vi "WzNetRem_Example_General.vi"() -> ()   [LabVIEW 2012]
uses:
  Wizzler_NetworkRemoteToolkit.lvlib
panel:
  out "Signal Goodness":cluster{"Value":dbl, "Warning":string} {"Value" scale=0.9..2.0}
  out "Signal Level":cluster{"Value":dbl, "Warning":string} {"Value" scale=0.0..65535.0}
  out "Time profile":cluster{"Time":dbl[], "Intensity":dbl[]}[](graph)
  out "Numerics":T1={"Autoco duration FWHM"=0.0, "FTL time width FWHM"=nan, "TBP FWHM"=nan, "Spectral width FWHM"=nan, "Time width FWHM"=nan, "Mean wavelength"=nan, "Time stand. dev."=nan, "FTL time stand. dev."=nan, "Mean freq"=nan, "Spectral stand. dev."=nan, "TBP stand. dev."=nan, "Spectral width FWHM - nu"=nan, "Spectral stand. dev. - nu"=nan} {"Spectral stand. dev. - nu" format="%#.1f"; "Spectral width FWHM - nu" format="%#.1f"; "TBP stand. dev." format="%#.3f"; "Spectral stand. dev." format="%#.1f"; "Mean freq" format="%#.1f"; "FTL time stand. dev." format="%#.1f"; "Time stand. dev." format="%#.1f"; "Mean wavelength" format="%#.1f"; "Time width FWHM" format="%#.1f"; "Spectral width FWHM" format="%#.1f"; "TBP FWHM" format="%#.3f"; "FTL time width FWHM" format="%#.1f"}
  in  "stop":bool
  in  "New Status":T2={"New Algorithm"=1, "Integration Time"=0.002, "LambdaMin"=7e-07, "LambdaMax"=9e-07} {"New Algorithm" items=["Spectrum", "SRSI"]}
  out "Previous Status":T3
  out "error out":errorcluster
  out "Time Stamp":string
  out "Spectral Data":cluster{"Frequencies":ext[], "Phase":dbl[]}[](graph)
  in  "machine name":string="127.0.0.1" caption="machine name (\"\":  open local reference)"
  in  "port number":u16=54321
  out "SerialID":string="Unknown"
  out "Software Version":string="Unknown"
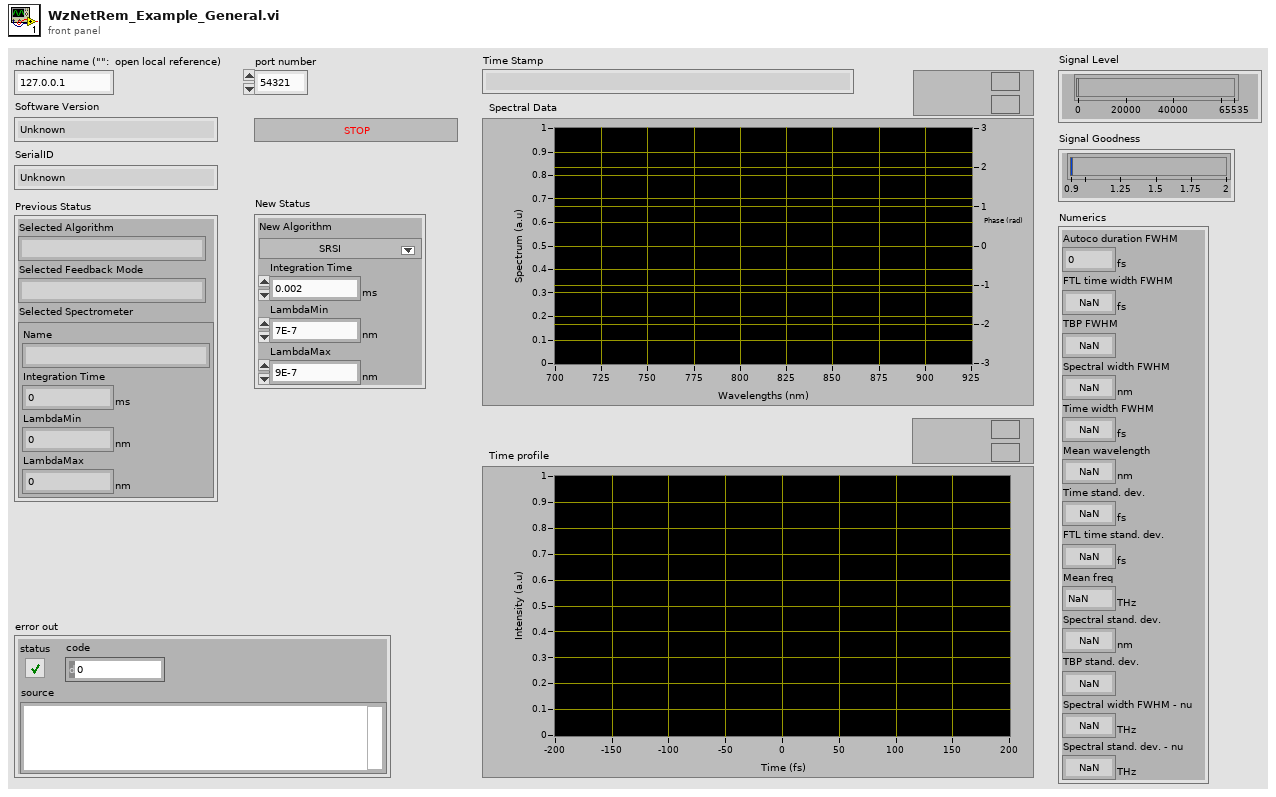
[diagram p1: front panel]
types:
  T1 = cluster{"Autoco duration FWHM":dbl[unit], "FTL time width FWHM":dbl[unit], "TBP FWHM":dbl, "Spectral width FWHM":dbl[unit], "Time width FWHM":dbl[unit], "Mean wavelength":dbl[unit], "Time stand. dev.":dbl[unit], "FTL time stand. dev.":dbl[unit], "Mean freq":dbl[unit], "Spectral stand. dev.":dbl[unit], "TBP stand. dev.":dbl, "Spectral width FWHM - nu":dbl[unit], "Spectral stand. dev. - nu":dbl[unit]}
  T2 = cluster{"New Algorithm":u16, "Integration Time":dbl[unit], "LambdaMin":sgl[unit], "LambdaMax":sgl[unit]}
  T3 = cluster{"Selected Algorithm":string, "Selected Feedback Mode":string, "Selected Spectrometer":cluster{"Name":string, "Integration Time":dbl[unit], "LambdaMin":sgl[unit], "LambdaMax":sgl[unit]}}
  T4 = cluster{"Name":string, "Integration Time":dbl[unit], "LambdaMin":sgl[unit], "LambdaMax":sgl[unit]}
  T5 = cluster{"Name":string, "Name":string, cluster{"Name":string, "Integration Time":dbl[unit], "LambdaMin":sgl[unit], "LambdaMax":sgl[unit]}}
  T6 = enum8{"Enabled", "Disabled", "Disabled and Grayed Out"}
  T7 = cluster{"Frequencies":dbl[], "Spectral Intensity":dbl[]}
  T8 = cluster{"Frequencies":dbl[], "Spectral Intensity":dbl[]}[]
  T9 = cluster{"Spectral profile":cluster{"Freq":dbl[], "Spectrum":dbl[], "Phase":dbl[], "Fit":dbl[], "Clipping mask":cluster{"start_index":i32, "width":i32}}, "Phase fit":cluster{"Ctrl freq":dbl[unit], "Poly. fit Coeffs.":dbl[]}, "Time profile":cluster{"Time":dbl[], "Intensity":dbl[], "Phase":dbl[]}, "Numerics":cluster{"Autoco duration FWHM":dbl[unit], "FTL time width FWHM":dbl[unit], "TBP FWHM":dbl, "Spectral width FWHM":dbl[unit], "Time width FWHM":dbl[unit], "Mean wavelength":dbl[unit], "Time stand. dev.":dbl[unit], "FTL time stand. dev.":dbl[unit], "Mean freq":dbl[unit], "Spectral stand. dev.":dbl[unit], "TBP stand. dev.":dbl, "Spectral width FWHM - nu":dbl[unit], "Spectral stand. dev. - nu":dbl[unit]}, "Time stamp":string, "Signal Quality":cluster{"Level":cluster{"Value":dbl, "String":string}, "Goodness":cluster{"Value":dbl, "String":string}, "Disable Num Displays":bool}}
  T10 = cluster{"Measured":cluster{"Time":dbl[], "Intensity":dbl[]}, "FTL":cluster{"Time":dbl[], "Intensity":dbl[]}}
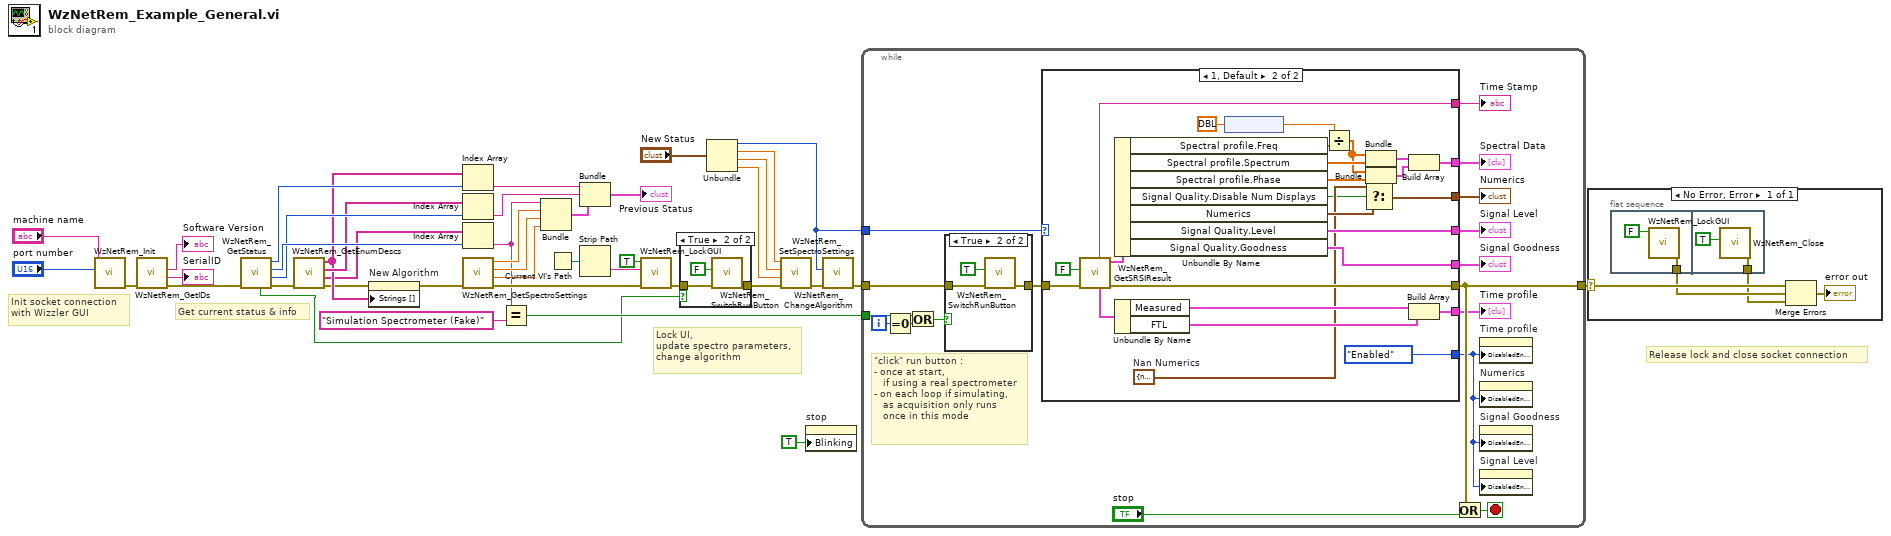
[diagram p0: block diagram]
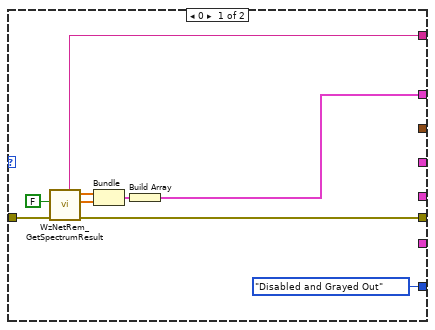
[diagram p3: hidden frame]
diagram:
  # "Init socket connection\nwith Wizzler GUI"
  # "Release lock and close socket connection"
  # "Lock UI, \nupdate spectro parameters,\nchange algorithm"
  # "Get current status & info"
  n1 = call "WzNetRem_Init.vi"("port number"="port number", "machine name"="machine name") -> ("error out"=w39:errorcluster)  [unwired: 9 in]
  n2 = call "WzNetRem_GetIDs.vi"("error in (no error)"=w39) -> ("error out"=w28:errorcluster, "SerialID"=→"SerialID":string, "Software Version"=→"Software Version":string)  [unwired: 8 in]
  n3 = call "WzNetRem_GetStatus.vi"("error in (no error)"=w28) -> ("error out"=w33:errorcluster, "Current Feedback Mode"=w30:i32, "Current Spectro Index"=w31:i32, "Current Algo Index"=w32:i32, "Running?"=w1:bool)  [unwired: 4 in, 2 out]
  n4 = call "WzNetRem_GetEnumDescs.vi"("error in"=w33) -> ("error out"=w18:errorcluster, "Spectrometers"=w8:string[], "Feedback Modes"=w29:string[], "Algorithms"=w20:string[])  [unwired: 7 in]
  n5 = property on="New Algorithm" class="Ring (strict)"(error in=w18, "Strings []"=w20) -> (error out=w17:errorcluster)  [unwired: 1 in, 1 out]
  n6 = Index Array(array=w20, index=w32) -> (element=w27:string)
  n7 = Index Array(array=w29, index=w30) -> (element=w26:string)
  n8 = Index Array(array=w8, index=w31) -> (element=w7:string)
  n9 = call "WzNetRem_GetSpectroSettings.vi"("error in (no error)"=w17) -> ("error out"=w19:errorcluster, "LambdaMax"=w23:sgl[unit], "LambdaMin"=w22:sgl[unit], "Integration Time"=w21:dbl[unit])  [unwired: 7 in]
  n10 = Equal?(x=w7, y="Simulation Spectrometer (Fake)" ("Name")) -> (x = y?=w5:bool)
  n11 = Bundle("Name"=w7, "Integration Time"=w21, "LambdaMin"=w22, "LambdaMax"=w23) -> (w24:T4)  [unwired: 1 in]
  n12 = Current VI's Path() -> (path=w35:path)
  n13 = Bundle("Name"=w27, "Name"=w26, w24) -> (→"Previous Status":T5)  [unwired: 1 in]
  n14 = Strip Path(path=w35) -> (name=w34:string)  [unwired: 1 out]
  n15 = call "WzNetRem_LockGUI.vi"("error in (no error)"=w19, "Locker ID"=w34, "Lock State"=TRUE) -> ("error out"=w15:errorcluster)  [unwired: 8 in]
  n16 = case shown="True" w1 {
    tunnel: w15 -> [w42 w44]
    tunnel: [w42 w43] -> w14
    frame False {
    }
    frame True {
      n17 = call "WzNetRem_SwitchRunButton.vi"("error in (no error)"=w44, "New Run State"=FALSE) -> ("error out"=w43:errorcluster)  [unwired: 9 in]
    }
  }
  n18 = Unbundle("New Status") -> ("New Algorithm"=w4:u16, "Integration Time"=w10:dbl[unit], "LambdaMin"=w11:sgl[unit], "LambdaMax"=w12:sgl[unit])
  n19 = call "WzNetRem_SetSpectroSettings.vi"("error in (no error)"=w14, "LambdaMax"=w12, "LambdaMin"=w11, "Integration Time"=w10) -> ("error out"=w9:errorcluster)  [unwired: 7 in]
  n20 = property on="stop" class="Bool"("Blinking"=TRUE) -> ()  [unwired: 2 in, 2 out]
  n21 = call "WzNetRem_ChangeAlgorithm.vi"("error in (no error)"=w9, "New Algo  Index"=w4) -> ("error out"=w16:errorcluster)  [unwired: 8 in, 1 out]
  n22 = while {
    tunnel: w16 -> [w62]
    tunnel: w5 -> [w56]
    tunnel: w4 -> [w54]
    tunnel: [w52] -> w3
    i -> [w58]
    stop <- w59 stop-if-true
    # "\"click\" run button :\n- once at start,\n   if using a real spectrometer\n- on each loop if simulating,\n   as acquisition only runs\n   once in this mode"
    n23 = Equal To 0?(x=w58) -> (x = 0?=w57:bool)
    n24 = Or(x=w56, y=w57) -> (x .or. y?=w55:bool)
    n25 = case shown="True" w55 {
      tunnel: w62 -> [w97 w100]
      tunnel: [w97 w98] -> w61
      frame False {
      }
      frame True {
        n26 = call "WzNetRem_SwitchRunButton.vi"("error in (no error)"=w100, "New Run State"=TRUE) -> ("error out"=w98:errorcluster)  [unwired: 9 in]
      }
    }
    n27 = case shown="1, Default" w54 {
      tunnel: w61 -> [w70 w95]
      tunnel: [w69 w94] -> w52
      tunnel: [w68 w93] -> w53
      tunnel: [_ w78] -> w51
      tunnel: [w64 w86] -> w50
      tunnel: [_ w84] -> w49
      tunnel: [T6."Disabled and Grayed Out" ("Disabled") T6."Enabled" ("Disabled")] -> w48
      tunnel: [_ w80] -> w47
      tunnel: [_ w79] -> w46
      frame 0 {
        n28 = call "WzNetRem_GetSpectrumResult.vi"("error in (no error)"=w70, "Ignore Old Results?"=FALSE ("Wait for next measurement?")) -> ("error out"=w69:errorcluster, "Spectral Intensity"=w66:dbl[], "Frequencies"=w67:dbl[], "Time Stamp"=w68:string)  [unwired: 6 in]
        n29 = Bundle("Frequencies"=w67, "Spectral Intensity"=w66) -> (w65:T7)  [unwired: 1 in]
        n30 = Build Array(w65) -> (w64:T8)
      }
      frame 1, Default {
        w76 = T1 {"Autoco duration FWHM"=nan, "FTL time width FWHM"=nan, "TBP FWHM"=nan, "Spectral width FWHM"=nan, "Time width FWHM"=nan, "Mean wavelength"=nan, "Time stand. dev."=nan, "FTL time stand. dev."=nan, "Mean freq"=nan, "Spectral stand. dev."=nan, "TBP stand. dev."=nan, "Spectral width FWHM - nu"=nan, "Spectral stand. dev. - nu"=nan}  # Nan Numerics
        n31 = call "WzNetRem_GetSRSIResult.vi"("error in (no error)"=w95, "Ignore Old Results?"=FALSE ("Wait for next measurement?")) -> ("error out"=w94:errorcluster, "Num Results"=w92:T9, "Time Intensities"=w85:T10, "Time Stamp"=w93:string)  [unwired: 4 in, 2 out]
        n32 = Unbundle By Name(w92) -> ("Spectral profile.Freq"=w90:dbl[], "Spectral profile.Spectrum"=w91:dbl[], "Spectral profile.Phase"=w89:dbl[], "Signal Quality.Disable Num Displays"=w72:bool, "Numerics"=w77:T1, "Signal Quality.Level"=w80:cluster{"Value":dbl, "String":string}, "Signal Quality.Goodness"=w79:cluster{"Value":dbl, "String":string})
        n33 = Unbundle By Name(w85) -> ("Measured"=w83:cluster{"Time":dbl[], "Intensity":dbl[]}, "FTL"=w82:cluster{"Time":dbl[], "Intensity":dbl[]})
        n34 = node(ext[unit] 299792458.0) -> (w73:ext)
        n35 = Divide(x=w73, y=w90) -> (x/y=w74:ext[])
        n36 = Select(t=w76, s=w72, f=w77) -> (s? t:f=w78:T1)
        n37 = Bundle(w74, "Spectrum"=w91) -> (w88:cluster{ext[], "Spectrum":dbl[]})  [unwired: 1 in]
        n38 = Bundle(w74, "Phase"=w89) -> (w87:cluster{ext[], "Phase":dbl[]})  [unwired: 1 in]
        n39 = Build Array(w88, w87) -> (w86:cluster{ext[], "Phase":dbl[]}[])
        n40 = Build Array(w83, w82) -> (w84:cluster{"Time":dbl[], "Intensity":dbl[]}[])
      }
    }
    "Time Stamp" <- w53
    "Spectral Data" <- w50
    "Numerics" <- w51
    "Time profile" <- w49
    "Signal Level" <- w47
    "Signal Goodness" <- w46
    n41 = Or(x=w52, y="stop") -> (x .or. y?=w59:bool)
    n42 = property on="Time profile" class="XYGraph (strict)"("DisabledEnum"=w48) -> ()  [unwired: 2 in, 2 out]
    n43 = property on="Numerics" class="Clust (strict)"("DisabledEnum"=w48) -> ()  [unwired: 2 in, 2 out]
    n44 = property on="Signal Goodness" class="Clust (strict)"("DisabledEnum"=w48) -> ()  [unwired: 2 in, 2 out]
    n45 = property on="Signal Level" class="Clust (strict)"("DisabledEnum"=w48) -> ()  [unwired: 2 in, 2 out]
  }
  n46 = case shown="No Error, Error" w3 {
    selector: w3 -> [w104]
    frame No Error {
      n47 = flat-sequence {
        tunnel: [w105] -> w102
        tunnel: [w108] -> w101
        frame #0 {
          n48 = call "WzNetRem_LockGUI.vi"("Lock State"=FALSE) -> ("error out"=w105:errorcluster)  [unwired: 10 in]
        }
        frame #1 {
          n49 = call "WzNetRem_Close.vi"("Force Meas. Stop"=TRUE) -> ("error out"=w108:errorcluster)  [unwired: 10 in]
        }
      }
      n50 = Merge Errors(w104, w102, w101) -> (→"error out":errorcluster)
    }
  }
